vi "Config Paths.vi"(7 "Create if Missing? (F)":bool, 8 "error in (no error)":errorcluster) -> (0 "error out":errorcluster, 1 "System Config Exists":bool, 2 "User Config Exists":bool, 3 "Paths":T1)   [LabVIEW 2020, in "PicoG-App.lvlib"]
uses:
  PicoG-App.lvlib
  Paths.ctl
  <vilib>/Utility/sysdir.llb/System Directory Type.ctl
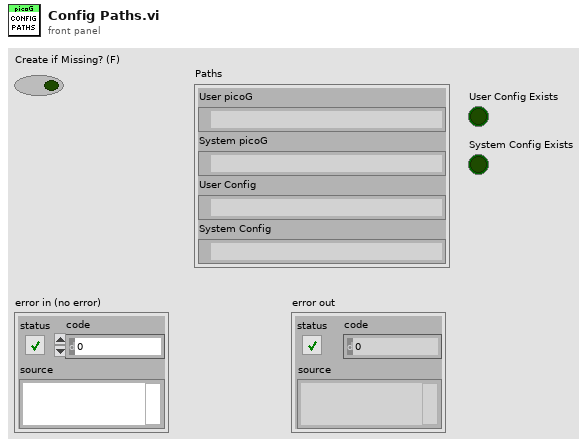
[diagram p1: front panel]
types:
  T1 = typedef "PicoG-App.lvlib/Paths.ctl" = cluster{"User picoG":path, "System picoG":path, "User Config":path, "System Config":path}
  T2 = typedef "System Directory Type.ctl" = i32
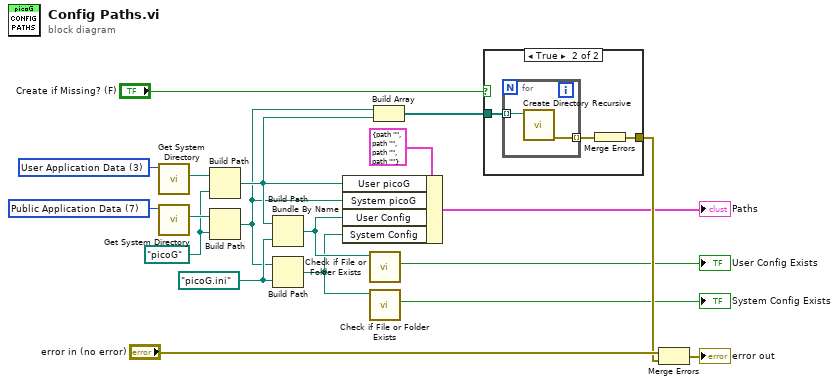
[diagram p0: block diagram]
diagram:
  w12 = path "picoG.ini" ("name or relative path")
  w15 = path "picoG" ("name or relative path")
  w18 = T2 7 items=["User Home"=0, "User Desktop"=1, "User Documents"=2, "User Application Data"=3, "User Preferences"=4, "User Temporary"=5, "Public Documents"=6, "Public Application Data"=7, "Public Preferences"=8, "Public Cache"=13, "System Core Libraries"=9, "System Installed Libraries"=10, "Application Files"=11, "Boot Volume Root"=12] ("system directory type")
  w19 = T2 3 items=["User Home"=0, "User Desktop"=1, "User Documents"=2, "User Application Data"=3, "User Preferences"=4, "User Temporary"=5, "Public Documents"=6, "Public Application Data"=7, "Public Preferences"=8, "Public Cache"=13, "System Core Libraries"=9, "System Installed Libraries"=10, "Application Files"=11, "Boot Volume Root"=12] ("system directory type")
  n1 = call <vilib>:"Get System Directory.vi"("system directory type"=w19) -> ("system directory"=w17:path)  [unwired: 10 in]
  n2 = call <vilib>:"Get System Directory.vi"("system directory type"=w18) -> ("system directory"=w16:path)  [unwired: 10 in]
  n3 = Build Path(base path=w17, name or relative path=w15) -> (appended path=w11:path)
  n4 = Build Path(base path=w16, name or relative path=w15) -> (appended path=w10:path)
  n5 = Build Path(base path=w11, name or relative path=w12) -> (appended path=w4:path)
  n6 = Build Path(base path=w10, name or relative path=w12) -> (appended path=w3:path)
  n7 = Bundle By Name(cluster=T1 {"User picoG"=path "", "System picoG"=path "", "User Config"=path "", "System Config"=path ""} ("Paths"), "User picoG"=w11, "System picoG"=w10, "User Config"=w4, "System Config"=w3) -> (→"Paths":T1)
  n8 = call <vilib>:"Check if File or Folder Exists.vi"("path"=w4) -> ("file or folder exists?"=→"User Config Exists":bool)  [unwired: 8 in, 2 out]
  n9 = call <vilib>:"Check if File or Folder Exists.vi"("path"=w3) -> ("file or folder exists?"=→"System Config Exists":bool)  [unwired: 8 in, 2 out]
  n10 = Build Array(w10, w11) -> (w9:path[])
  n11 = case shown="True" "Create if Missing? (F)" {
    tunnel: w9 -> [_ w22]
    tunnel: [_ w20] -> w7
    frame False {
    }
    frame True {
      n12 = for {
        tunnel: w22 -> [w24] mode=indexing
        tunnel: [w23] -> w21 mode=indexing
        n13 = call <vilib>:"Create Directory Recursive.vi"("directory"=w24) -> ("error out"=w23:errorcluster)  [unwired: 4 in, 2 out]
      }
      n14 = Merge Errors(w21) -> (w20:errorcluster)
    }
  }
  n15 = Merge Errors("error in (no error)", w7) -> (→"error out":errorcluster)
